vi "ReadImageDataFromMap.vi"(7 "map":T1, 8 "error in (no error)":errorcluster) -> (0 "error out":errorcluster, 1 "image height":i32, 2 "image width":i32, 3 "image data":sgl[](array[numeric]), 4 "image status":string, 5 "map out":T1, 6 "image timestamp":timestamp)   [LabVIEW 2017]
uses:
  <vilib>/addons/PointValueMap/controls/PointMap.ctl
  <vilib>/addons/PointValueMap/subVIs/Point_Read_variant.vi
  <vilib>/addons/PointValueMap/subVIs/Point_Read_i32.vi
  <vilib>/addons/PointValueMap/subVIs/Point_Read_string.vi
  <vilib>/addons/PointValueMap/PointValueMap.lvlib
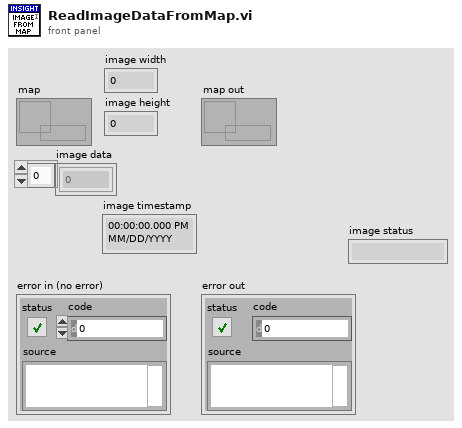
[diagram p1: front panel]
types:
  T1 = typedef "PointValueMap.lvlib/PointMap.ctl" = refnum<data-value>
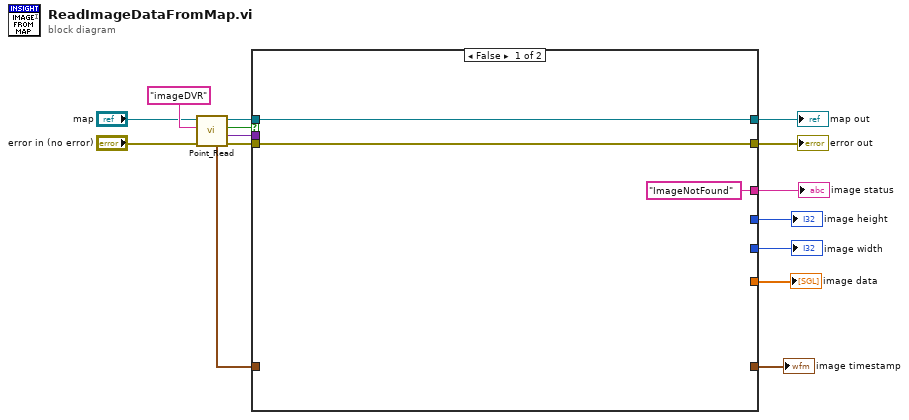
[diagram p0: block diagram]
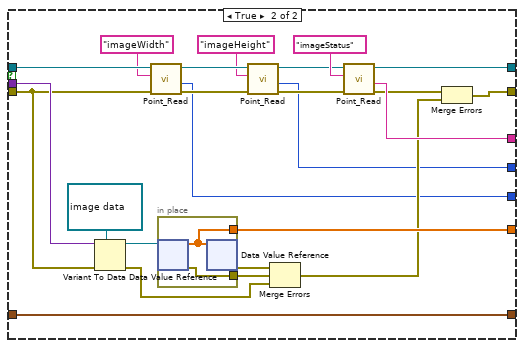
[diagram p2: hidden frame]
diagram:
  n1 = call-poly <vilib>:"Point_Read.vi"("Error In"="error in (no error)", "Tag"="imageDVR", "Map"="map") -> ("Error Out"=w10:errorcluster, "Value"=w7:variant, "Found?"=w8:bool, "Map Out"=w11:T1, "Time Stamp"=w5:timestamp)  [unwired: 3 in, 1 out]
  n2 = case shown="False" w8 {
    tunnel: [w18 w42] -> w13
    tunnel: [w17 w22] -> w12
    tunnel: w11 -> [w18 w40]
    tunnel: w10 -> [w17 w32]
    tunnel: w7 -> [_ w33]
    tunnel: [_ w29] -> w6
    tunnel: [_ w25] -> w4
    tunnel: w5 -> [_ w25]
    tunnel: ["ImageNotFound" ("Value") w24] -> w3
    tunnel: [_ w20] -> w2
    tunnel: [_ w19] -> w1
    frame False {
    }
    frame True {
      n3 = Variant To Data(error in=w32, type=refnum<data-value> refnum ("data value reference"), Variant=w33) -> (data=w30:refnum<data-value>, error out=w26:errorcluster)
      n4 = call-poly <vilib>:"Point_Read.vi"("Error In"=w32, "Tag"="imageWidth", "Map"=w40) -> ("Error Out"=w35:errorcluster, "Value"=w20:i32, "Map Out"=w39:T1)  [unwired: 3 in, 3 out]
      n5 = in-place {
        in-place-border: [w43] -> w29
        in-place-border: [w44] -> w27
        n6 = in-place-dvr #1(w30) -> (w43:sgl[], w44:errorcluster)
        n7 = in-place-dvr #1(w43) -> (w28:errorcluster)  [unwired: 1 out]
      }
      n8 = call-poly <vilib>:"Point_Read.vi"("Error In"=w35, "Tag"="imageHeight", "Map"=w39) -> ("Error Out"=w34:errorcluster, "Value"=w19:i32, "Map Out"=w38:T1)  [unwired: 3 in, 3 out]
      n9 = Merge Errors(w28, w27, w26) -> (w21:errorcluster)
      n10 = call-poly <vilib>:"Point_Read.vi"("Error In"=w34, "Tag"="imageStatus", "Map"=w38) -> ("Error Out"=w23:errorcluster, "Value"=w24:string, "Map Out"=w42:T1)  [unwired: 3 in, 3 out]
      n11 = Merge Errors(w23, w21) -> (w22:errorcluster)
    }
  }
  "map out" <- w13
  "error out" <- w12
  "image data" <- w6
  "image width" <- w2
  "image height" <- w1
  "image timestamp" <- w4
  "image status" <- w3
